vi "User Controls.vi"() -> ()   [LabVIEW 2015]
panel:
  in  "Short":bool
  out "Wire Length Out":dbl
  in  "Short Wire Length (mm)":dbl
  in  "Long Wire Length (mm)":dbl
  out "Has measured?":bool=TRUE
  out "Nth Measurement":i32
  out "t < X ?":bool
  in  "Get Tension":bool
  in  "Record":bool
  out "DAQ":dbl
  out "Charge time(s)":dbl caption="Elapsed Time (s)"
  in  "Charge Time (s)":dbl
  out "charging":bool
  # "Outputs"
  # "Inputs"
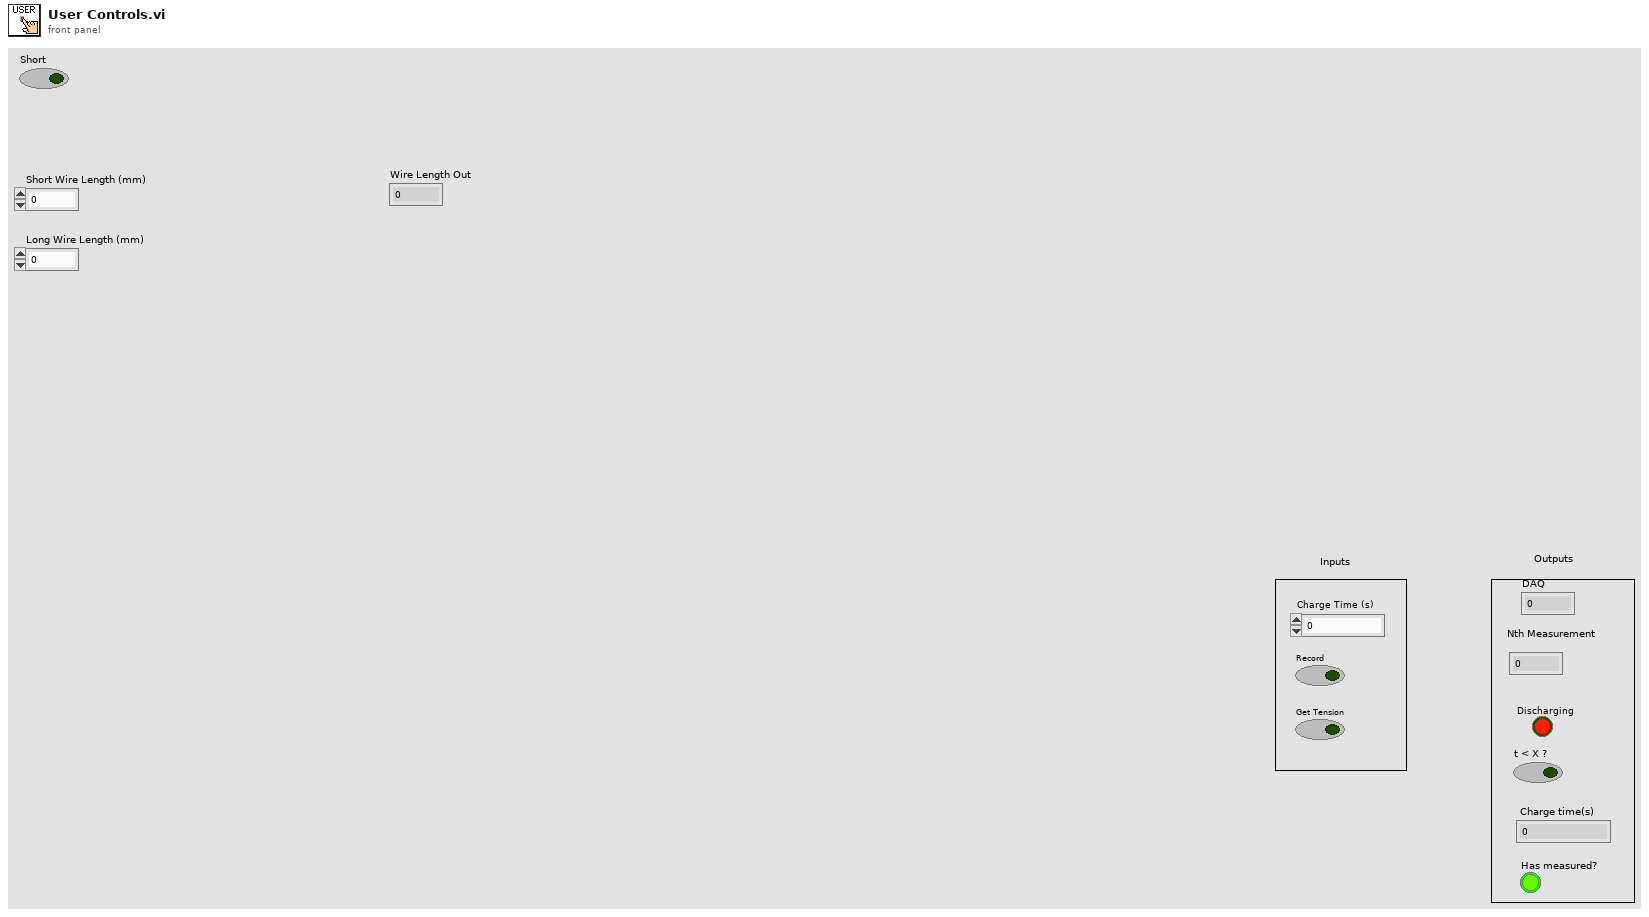
[diagram p1: front panel]
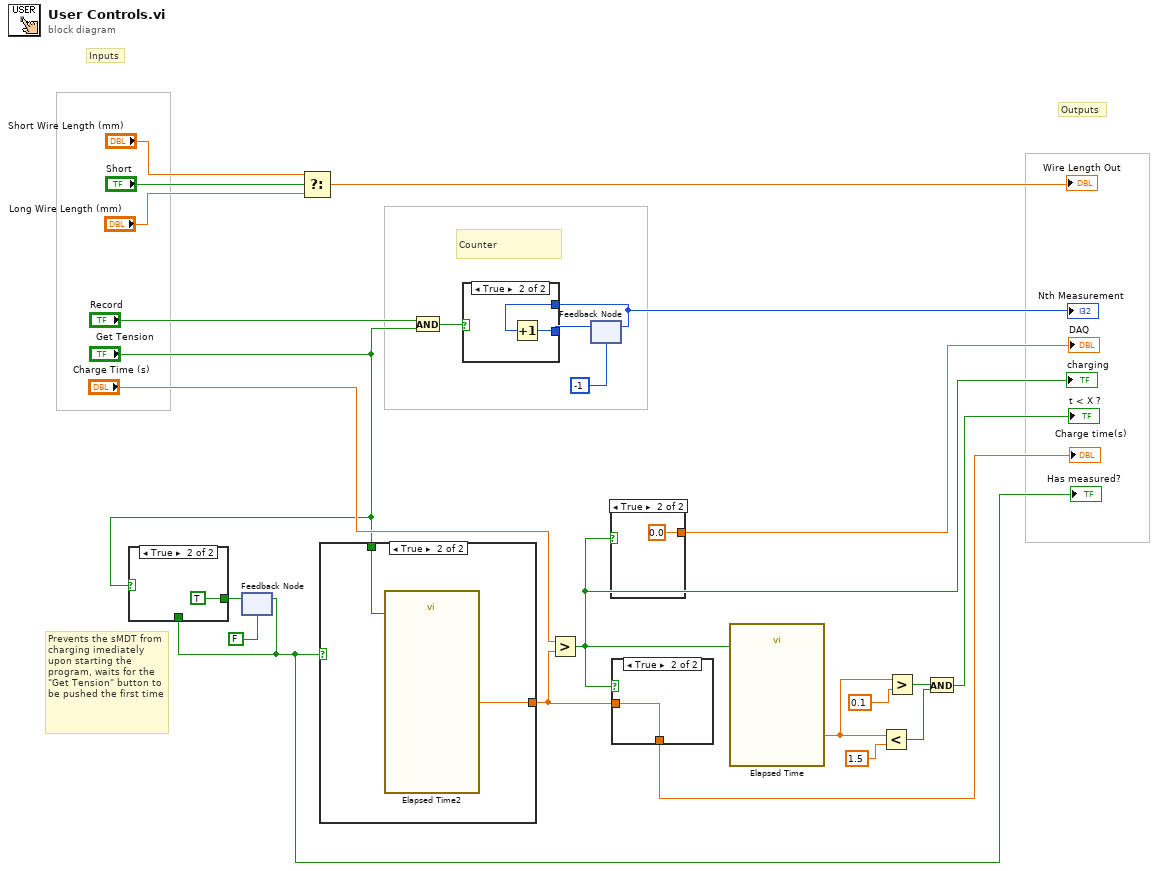
[diagram p0: block diagram]
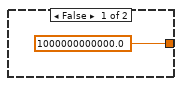
[diagram p3: hidden frame]
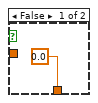
[diagram p4: hidden frame]
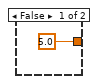
[diagram p6: hidden frame]
diagram:
  # "Prevents the sMDT from charging imediately upon starting the program, waits for the \"Get Tension\" button to be pushed the first time"
  # "Outputs"
  # "Inputs"
  # "Counter"
  n1 = feedback #1(FALSE) -> (w5:bool)
  "Has measured?" <- w5
  n2 = case shown="True" "Get Tension" {
    tunnel: [w25 TRUE] -> w9
    tunnel: w5 -> [w25 _]
    frame False {
    }
    frame True {
    }
  }
  n3 = feedback-in #1(w9) -> ()
  n4 = Select(t="Short Wire Length (mm)", s="Short", f="Long Wire Length (mm)") -> (s? t:f=→"Wire Length Out":dbl)
  n5 = case shown="True" w5 {
    tunnel: "Get Tension" -> [_ w29]
    tunnel: [1000000000000.0 w28] -> w6
    frame False {
    }
    frame True {
      n6 = call "Elapsed Time2"("Reset"=w29) -> ("Elapsed Time (s)"=w28:dbl)  [unwired: 11 in, 7 out]
    }
  }
  n7 = And(x="Record", y="Get Tension") -> (x .and. y?=w23:bool)
  n8 = Greater?(x="Charge Time (s)", y=w6) -> (0:w10:bool)
  "charging" <- w10
  n9 = feedback #2(-1) -> (w22:i32)
  "Nth Measurement" <- w22
  n10 = case shown="True" w23 {
    tunnel: [w30 w32] -> w17
    tunnel: w22 -> [w30 w31]
    frame False {
    }
    frame True {
      n11 = Increment(x=w31) -> (x+1=w32:i32)
    }
  }
  n12 = feedback-in #2(w17) -> ()
  n13 = case shown="True" w10 {
    tunnel: [5.0 0.0] -> w21
    frame False {
    }
    frame True {
    }
  }
  "DAQ" <- w21
  n14 = case shown="True" w10 {
    tunnel: w6 -> [_ w36]
    tunnel: [0.0 w36] -> w20
    frame False {
    }
    frame True {
    }
  }
  "Charge time(s)" <- w20
  n15 = call "Elapsed Time"("Reset"=w10) -> ("Elapsed Time (s)"=w11:dbl)  [unwired: 11 in, 7 out]
  n16 = Less?(x=w11, y=1.5) -> (x < y?=w14:bool)
  n17 = Greater?(x=w11, y=0.1) -> (0:w15:bool)
  n18 = And(x=w15, y=w14) -> (x .and. y?=→"t < X ?":bool)
